vi "Periodic Tasks.vi"(8 "error in":errorcluster) -> ()   [LabVIEW 2020]
doc: "This VI runs in parallel to other tasks. It can contain as many user-defined periodic loops as you need. These can carry out PID or other sorts of timed response."
uses:
  <vilib>/Rock Robotics/WPI/Joystick/XBox Buttons Indexer.ctl
  <vilib>/Rock Robotics/WPI/ThirdParty/JAS_Junk/TrajLib/SlewRateLimiter_New.vi
  <vilib>/Rock Robotics/WPI/ThirdParty/JAS_Junk/TrajLib/SlewRateLimiter_Reset.vi
  <vilib>/Rock Robotics/WPI/ThirdParty/JAS_Junk/TrajLib/SlewRateLimiter_Calculate.vi
  <vilib>/Rock Robotics/WPI/ThirdParty/JAS_Junk/TrajLib/SlewRateLimiter_SetRate.vi
  <vilib>/Rock Robotics/WPI/Utilities/WPI_GetSetVariantRefNum.vi
  Robot Global Data.vi
  <vilib>/Rock Robotics/Network Tables/NT Write Number.vi
  <vilib>/Rock Robotics/WPI/ThirdParty/JAS_Junk/TrajLib/Trajectory_Library.lvlib
panel:
  out "limit 5":bool
  out "limit 4":bool
  out "limit 3":bool
  out "limit 2":bool
  out "limit 1":bool
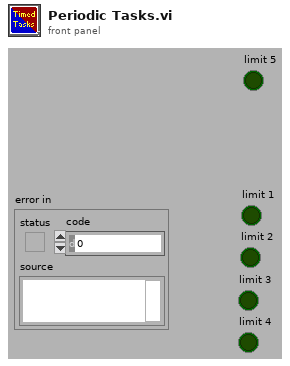
[diagram p1: front panel]
types:
  T1 = typedef "WPI_MotorControlDeviceRef.ctl" = cluster{"DeviceStatus":errorcluster, "Type":T2, "PWM":cluster{"PWM Channel":T3, "DeadBand":T4}, "CAN":cluster{"Device Number":u8, "SetOutput VI Ref":variant, "GetOutput VI Ref":variant, "Enable VI Ref":variant, "Disable VI Ref":variant, "Data":variant}, "Invert":bool, "DIO PWM":cluster{"PWM \"Enable\" Channel":T3, "DIOChannel":T5, "PWM Rate":dbl}}
  T2 = typedef "WPI_MotorControlType.ctl" = enum16{"PWM", "CAN", "DIO PWM"}
  T3 = typedef "FPGA_DIOPWMChannel.ctl" = enum8{"PWM 0", "PWM 1", "PWM 2", "PWM 3", "PWM 4", "PWM 5", "PWM 6", "PWM 7", "PWM 8", "PWM 9", "PWM MXP 0", "PWM MXP 1", "PWM MXP 2", "PWM MXP 3", "PWM MXP 4", "PWM MXP 5", "PWM MXP 6", "PWM MXP 7", "PWM MXP 8", "PWM MXP 9", "Invalid"}
  T4 = typedef "WPI_PWMDeadband.ctl" = cluster{"Name":string, "maxPositivePwm":i32, "minPositivePwm":i32, "centerPwm":i32, "maxNegativePwm":i32, "minNegativePwm":i32, "angularRange":u16}
  T5 = typedef "FPGA_DIOChannel.ctl" = enum8{"DIO 0", "DIO 1", "DIO 2", "DIO 3", "DIO 4", "DIO 5", "DIO 6", "DIO 7", "DIO 8", "DIO 9", "DIO MXP 0", "DIO MXP 1", "DIO MXP 2", "DIO MXP 3", "DIO MXP 4", "DIO MXP 5", "DIO MXP 6", "DIO MXP 7", "DIO MXP 8", "DIO MXP 9", "DIO MXP 10", "DIO MXP 11", "DIO MXP 12", "DIO MXP 13", "DIO MXP 14", "DIO MXP 15", "SPI Port CS1", "SPI Port CS2", "SPI Port CS3", "SPI Port MISO", "SPI Port MOSI", "Invalid"}
  T6 = typedef "WPI_SwitchDevRef.ctl" = cluster{"DevStatus":errorcluster, "DIO Channel":T5, "CntIndex":T7, "Normally Closed":bool}
  T7 = typedef "FPGA_CounterCtrSystemIndex.ctl" = enum8{"Ctr 0", "Ctr 1", "Ctr 2", "Ctr 3", "Ctr 4", "Ctr 5", "Ctr 6", "Ctr 7", "Invalid"}
  T8 = typedef "WPI_GyroDevRef.ctl" = cluster{"DevStatus":errorcluster, "Analog Channel":T9, "Gain (VoltsPerDegree/Second)":dbl, "Gyro Type":enum16{"Analog", "XRS450"}, "Handle":i32, "SPI Bus":T10, "Device Found":bool, "Sample Rate":dbl, "Calibrate On Open":bool, "Offset":dbl}
  T9 = typedef "FPGA_AIChannel.ctl" = enum8{"AI 0", "AI 1", "AI 2", "AI 3", "AI MXP 0", "AI MXP 1", "AI MXP 2", "AI MXP 3", "Invalid"}
  T10 = typedef "spi_bus.ctl" = enum16{"SPI On-Board, CS0", "SPI On-Board, CS1", "SPI On-Board, CS2", "SPI On-Board, CS3", "SPI MXP", "Invalid"}
  T11 = typedef "XBox Buttons Indexer.ctl" = enum16{"A", "B", "X", "Y", "Left Bumper", "Right Bumper", "Back", "Start", "Left Joystick", "Right Joystick"}
  T12 = typedef "Trajectory_Library.lvlib/SWERVE_DRIVE_MODULE_STATE.ctl" = cluster{"Speed":dbl, "Angle":T13}
  T13 = typedef "Trajectory_Library.lvlib/ROTATION2D.ctl" = cluster{"VALUE":dbl, "COS":dbl, "SIN":dbl}
  T14 = typedef "WPI_JoystickDevRef.ctl" = cluster{"Device":T15}
  T15 = typedef "WPI_JoystickDeviceEnum.ctl" = enum16{"USB 0", "USB 1", "USB 2", "USB 3", "USB 4", "USB 5"}
  T16 = typedef "Trajectory_Library.lvlib/SWERVE_DRIVE_MODULE_POSITION.ctl" = cluster{"Distance":dbl, "Angle":T13, "P":bool}
  T17 = typedef "WPI_DriverStationRobotMode2.ctl" = enum16{"Autonomous Disabled", "Autonomous Enabled", "Teleop Disabled", "Teleop Enabled", "Disconnected", "Finish", "Test Disabled", "Test Enabled", "Emergency Stopped"}
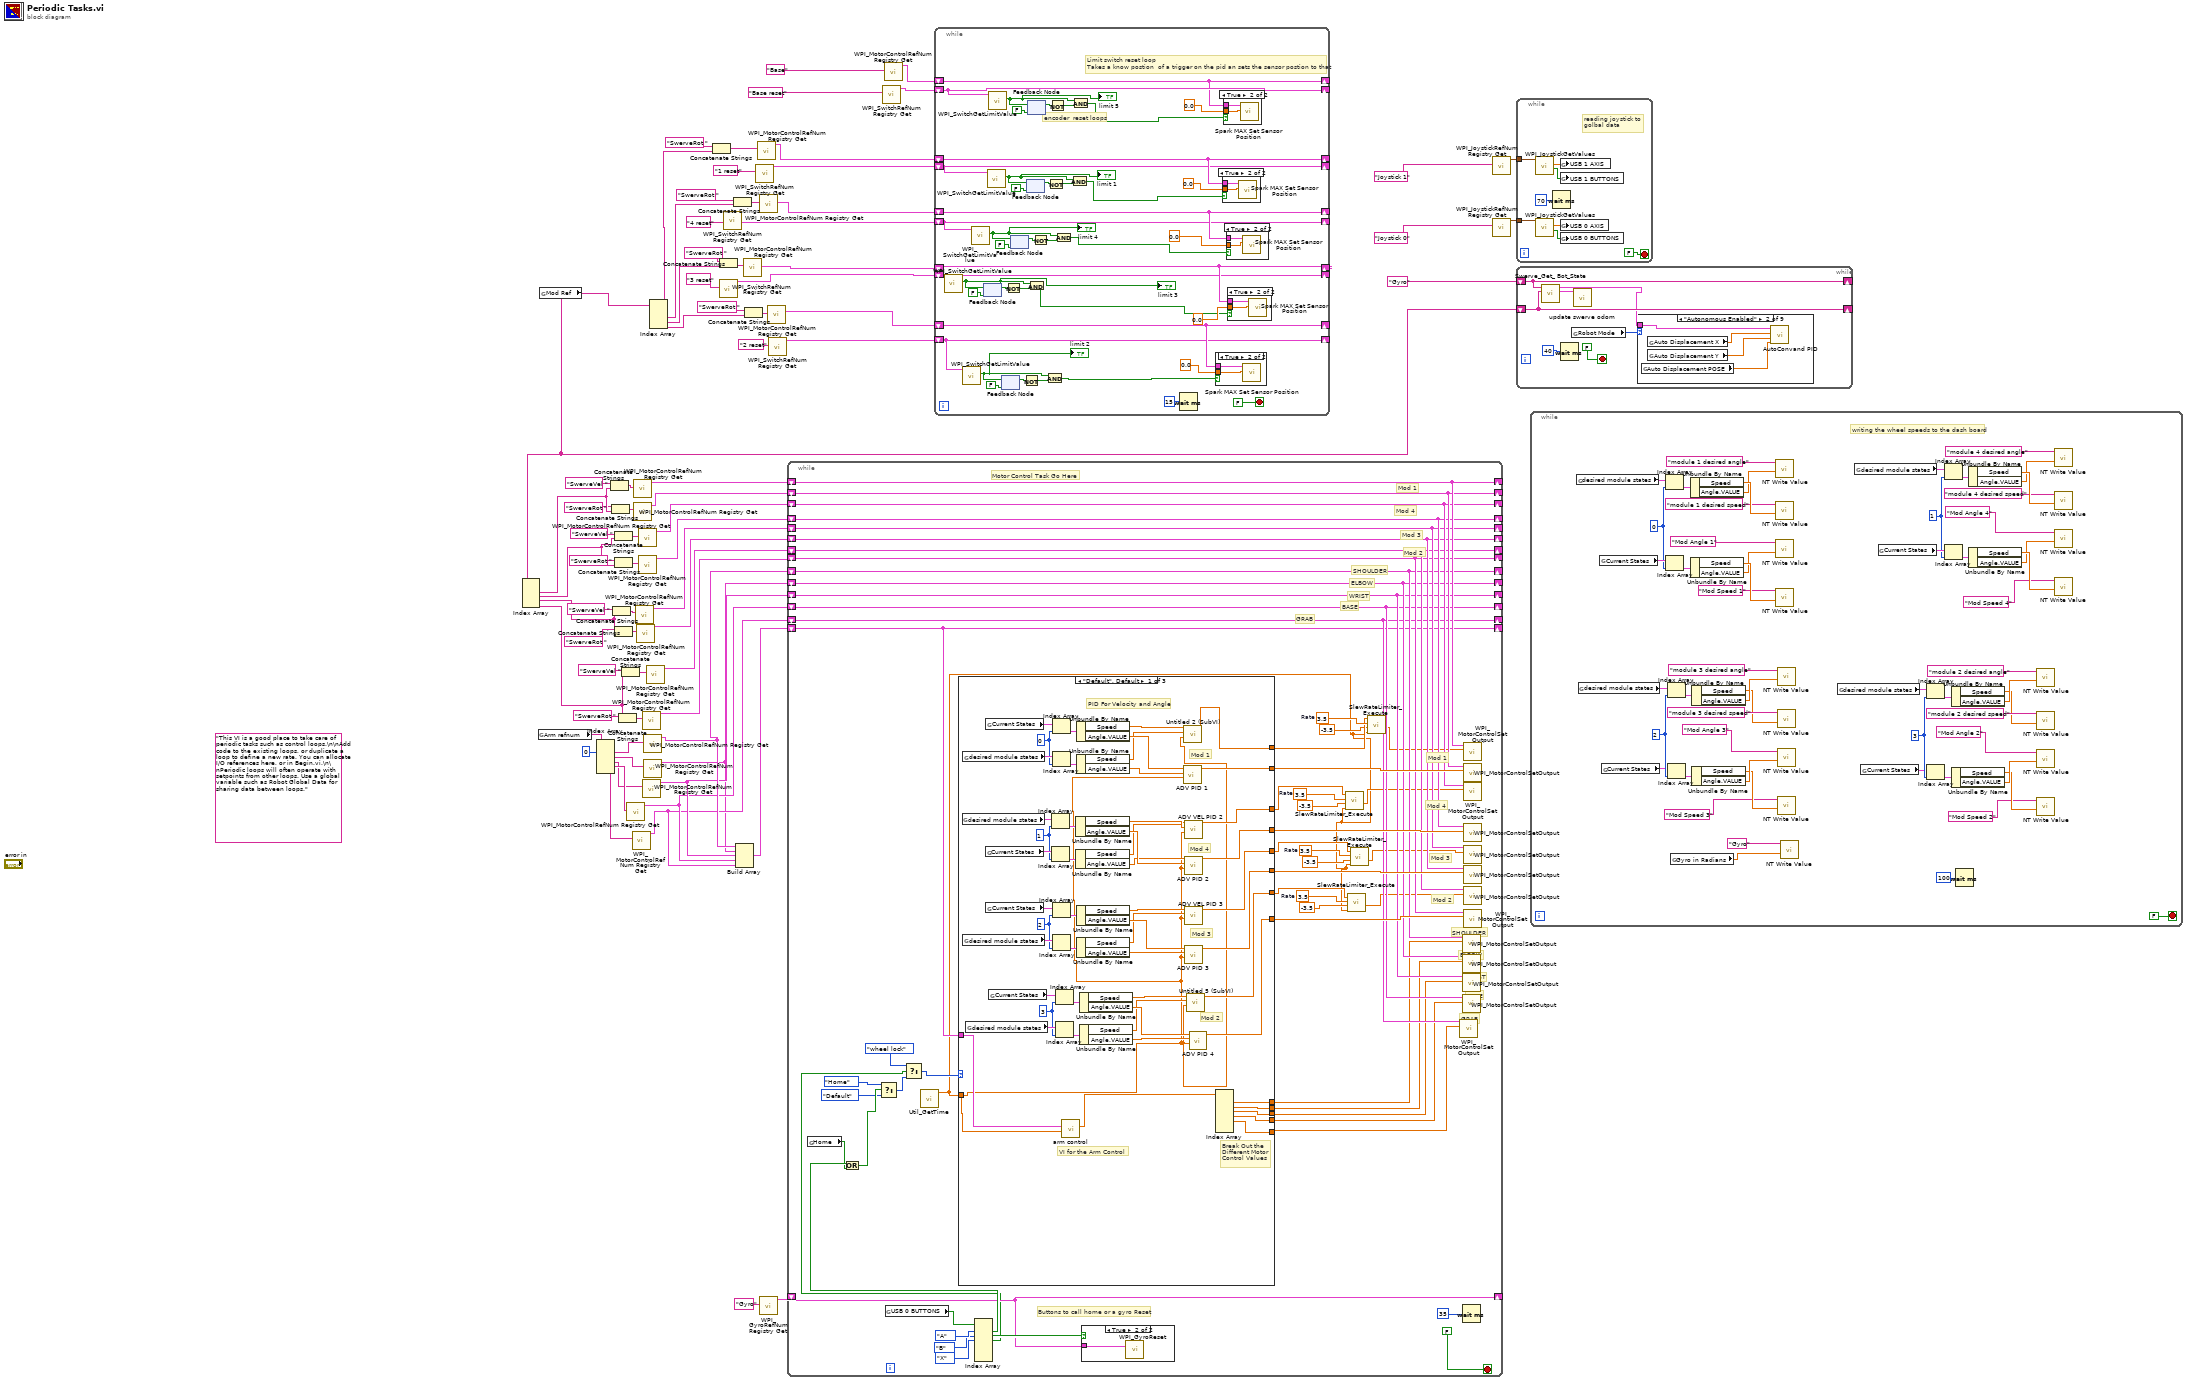
[diagram p0: block diagram]
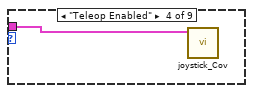
[diagram p4: hidden frame]
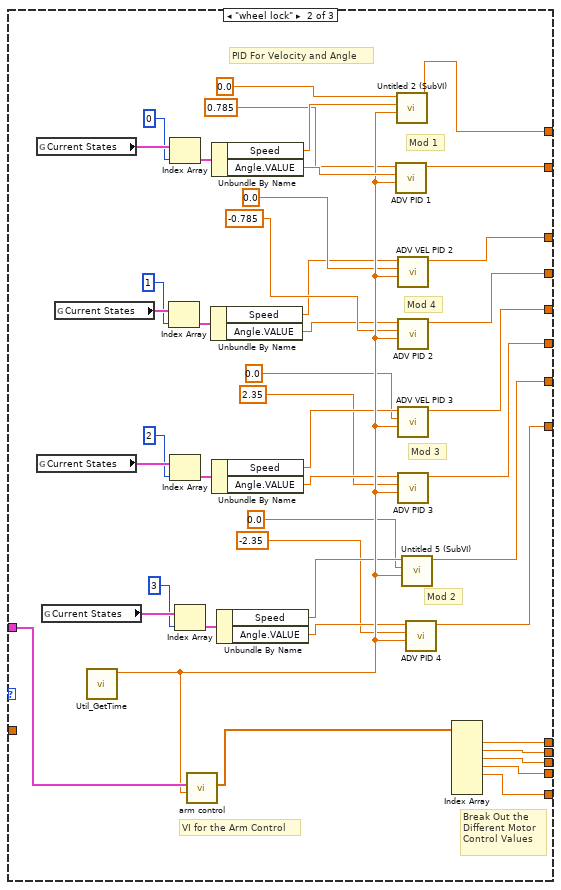
[diagram p10: hidden frame]
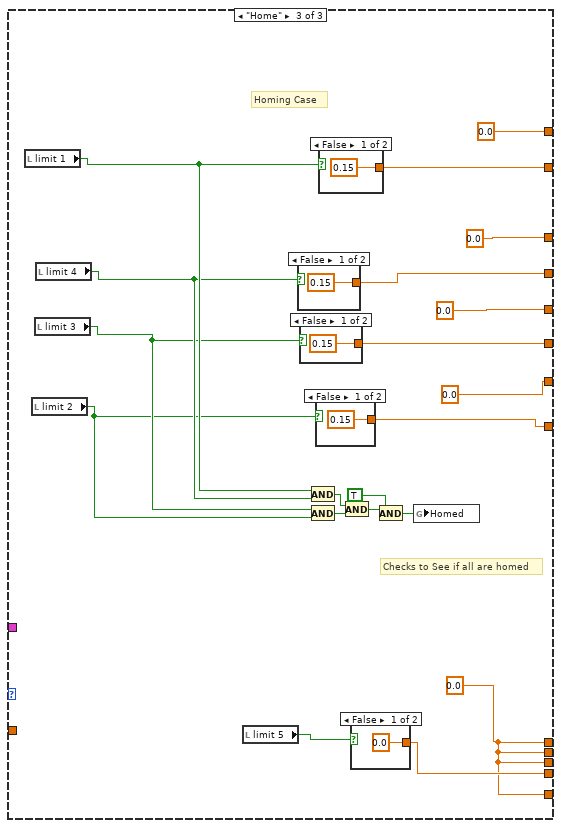
[diagram p11: hidden frame]
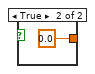
[diagram p12: hidden frame]
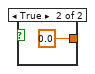
[diagram p13: hidden frame]
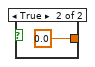
[diagram p14: hidden frame]
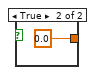
[diagram p15: hidden frame]
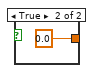
[diagram p16: hidden frame]
diagram:
  (unwired) "This VI is a good place to take care of periodic tasks such as control loops.\n\nAdd code to the existing loops, or duplicate a loop to define a new rate. You can allocate I/O references here, or in Begin.vi.\n\nPeriodic loops will often operate with setpoints from other loops. Use a global variable such as Robot Global Data for sharing data between loops."
  n1 = global read "Robot Global Data.vi" "Arm refnum"() -> (w7:string[])
  n2 = global read "Robot Global Data.vi" "Mod Ref"() -> (w22:string[])
  n3 = Index Array(array=w22) -> (element #1=w35:string, element #2=w40:string, element #3=w49:string, element #4=w50:string)  [unwired: 4 in]
  n4 = Index Array(array=w7, index #1=0 ("index")) -> (element #1=w9:string, element #2=w10:string, element #3=w11:string, element #4=w12:string, element #5=w13:string)  [unwired: 4 in]
  n5 = Concatenate Strings("SwerveVel " ("refnum name"), w35) -> (w32:string)
  n6 = Concatenate Strings("SwerveRot " ("refnum name"), w35) -> (w31:string)
  n7 = Concatenate Strings("SwerveVel " ("refnum name"), w49) -> (w42:string)
  n8 = Concatenate Strings("SwerveVel " ("refnum name"), w40) -> (w38:string)
  n9 = Concatenate Strings("SwerveRot " ("refnum name"), w40) -> (w39:string)
  n10 = Concatenate Strings("SwerveRot " ("refnum name"), w49) -> (w41:string)
  n11 = Concatenate Strings("SwerveRot " ("refnum name"), w50) -> (w48:string)
  n12 = Concatenate Strings("SwerveVel " ("refnum name"), w50) -> (w47:string)
  n13 = call <vilib>:"WPI_MotorControlRefNum Registry Get.vi"("refnum name"=w12) -> ("MotorControlDevRef"=w4:T1)  [unwired: 9 in, 1 out]
  n14 = call <vilib>:"WPI_MotorControlRefNum Registry Get.vi"("refnum name"=w13) -> ("MotorControlDevRef"=w3:T1)  [unwired: 9 in, 1 out]
  n15 = call <vilib>:"WPI_MotorControlRefNum Registry Get.vi"("refnum name"=w32) -> ("MotorControlDevRef"=w30:T1)  [unwired: 9 in, 1 out]
  n16 = call <vilib>:"WPI_MotorControlRefNum Registry Get.vi"("refnum name"=w31) -> ("MotorControlDevRef"=w29:T1)  [unwired: 9 in, 1 out]
  n17 = call <vilib>:"WPI_MotorControlRefNum Registry Get.vi"("refnum name"=w42) -> ("MotorControlDevRef"=w26:T1)  [unwired: 9 in, 1 out]
  n18 = call <vilib>:"WPI_MotorControlRefNum Registry Get.vi"("refnum name"=w41) -> ("MotorControlDevRef"=w25:T1)  [unwired: 9 in, 1 out]
  n19 = call <vilib>:"WPI_MotorControlRefNum Registry Get.vi"("refnum name"=w38) -> ("MotorControlDevRef"=w28:T1)  [unwired: 9 in, 1 out]
  n20 = call <vilib>:"WPI_MotorControlRefNum Registry Get.vi"("refnum name"=w39) -> ("MotorControlDevRef"=w27:T1)  [unwired: 9 in, 1 out]
  n21 = call <vilib>:"WPI_MotorControlRefNum Registry Get.vi"("refnum name"=w48) -> ("MotorControlDevRef"=w23:T1)  [unwired: 9 in, 1 out]
  n22 = call <vilib>:"WPI_MotorControlRefNum Registry Get.vi"("refnum name"=w11) -> ("MotorControlDevRef"=w5:T1)  [unwired: 9 in, 1 out]
  n23 = call <vilib>:"WPI_MotorControlRefNum Registry Get.vi"("refnum name"=w9) -> ("MotorControlDevRef"=w6:T1)  [unwired: 9 in, 1 out]
  n24 = call <vilib>:"WPI_MotorControlRefNum Registry Get.vi"("refnum name"=w10) -> ("MotorControlDevRef"=w2:T1)  [unwired: 9 in, 1 out]
  n25 = call <vilib>:"WPI_MotorControlRefNum Registry Get.vi"("refnum name"=w47) -> ("MotorControlDevRef"=w24:T1)  [unwired: 9 in, 1 out]
  n26 = Index Array(array=w22) -> (element #1=w65:string, element #2=w61:string, element #3=w58:string, element #4=w55:string)  [unwired: 4 in]
  n27 = Concatenate Strings("SwerveRot " ("refnum name"), w65) -> (w64:string)
  n28 = call <vilib>:"WPI_SwitchRefNum Registry Get.vi"("refnum name"="3 reset") -> ("SwitchDevRef"=w72:T6)  [unwired: 9 in, 1 out]
  n29 = Concatenate Strings("SwerveRot " ("refnum name"), w58) -> (w57:string)
  n30 = call <vilib>:"WPI_SwitchRefNum Registry Get.vi"("refnum name"="4 reset") -> ("SwitchDevRef"=w71:T6)  [unwired: 9 in, 1 out]
  n31 = Concatenate Strings("SwerveRot " ("refnum name"), w61) -> (w60:string)
  n32 = Build Array(w6, w2, w5, w4, w3) -> (w1:T1[])
  n33 = call <vilib>:"WPI_MotorControlRefNum Registry Get.vi"("refnum name"=w57) -> ("MotorControlDevRef"=w73:T1)  [unwired: 9 in, 1 out]
  n34 = Concatenate Strings("SwerveRot " ("refnum name"), w55) -> (w54:string)
  n35 = call <vilib>:"WPI_SwitchRefNum Registry Get.vi"("refnum name"="1 reset") -> ("SwitchDevRef"=w66:T6)  [unwired: 9 in, 1 out]
  n36 = call <vilib>:"WPI_MotorControlRefNum Registry Get.vi"("refnum name"=w64) -> ("MotorControlDevRef"=w67:T1)  [unwired: 9 in, 1 out]
  n37 = call <vilib>:"WPI_MotorControlRefNum Registry Get.vi"("refnum name"=w60) -> ("MotorControlDevRef"=w70:T1)  [unwired: 9 in, 1 out]
  n38 = call <vilib>:"WPI_GyroRefNum Registry Get.vi"("refnum name"="Gyro") -> ("GyroDevRef"=w52:T8)  [unwired: 9 in, 1 out]
  n39 = call <vilib>:"WPI_MotorControlRefNum Registry Get.vi"("refnum name"=w54) -> ("MotorControlDevRef"=w76:T1)  [unwired: 9 in, 1 out]
  n40 = call <vilib>:"WPI_SwitchRefNum Registry Get.vi"("refnum name"="2 reset") -> ("SwitchDevRef"=w77:T6)  [unwired: 9 in, 1 out]
  n41 = while {
    shift-right: [w124] -> _
    shift-left: w30 -> [w124]
    shift-right: [w123] -> _
    shift-left: w29 -> [w123]
    shift-right: [w122] -> _
    shift-left: w28 -> [w122]
    shift-right: [w121] -> _
    shift-left: w27 -> [w121]
    shift-right: [w120] -> _
    shift-left: w26 -> [w120]
    shift-right: [w119] -> _
    shift-left: w25 -> [w119]
    shift-right: [w118] -> _
    shift-left: w24 -> [w118]
    shift-right: [w117] -> _
    shift-left: w23 -> [w117]
    shift-right: [w116] -> _
    shift-left: w52 -> [w116]
    shift-right: [w113] -> _
    shift-left: w6 -> [w113]
    shift-right: [w112] -> _
    shift-left: w2 -> [w112]
    shift-right: [w111] -> _
    shift-left: w5 -> [w111]
    shift-right: [w110] -> _
    shift-left: w4 -> [w110]
    shift-right: [w109] -> _
    shift-left: w3 -> [w109]
    shift-right: [w108] -> _
    shift-left: w1 -> [w108]
    stop <- FALSE stop-if-true
    w82 = 3.5  # Rate
    w86 = 3.5  # Rate
    w89 = 3.5  # Rate
    w94 = 3.5  # Rate
    # "Buttons to call home or a gyro Reset"
    # "Mod 4"
    # "Mod 4"
    # "Mod 3"
    # "Mod 3"
    # "Mod 2"
    # "Mod 2"
    # "Mod 1"
    # "Mod 1"
    # "GRAB"
    # "BASE"
    # "WRIST"
    # "ELBOW"
    # "SHOULDER"
    # "BASE"
    # "GRAB"
    # "WRIST"
    # "ELBOW"
    # "SHOULDER"
    # "Motor Control Task Go Here"
    n42 = global read "Robot Global Data.vi" "Home"() -> (w115:bool)
    n43 = global read "Robot Global Data.vi" "USB 0 BUTTONS"() -> (w114:bool[])
    n44 = call <vilib>:"Util_GetTime.vi"() -> ("FPGA_Time_Seconds"=w78:dbl)  [unwired: 9 in, 2 out]
    n45 = Index Array(array=w114, index #1=XBox_Buttons_Indexer."A" ("XBox Buttons"), index #2=XBox_Buttons_Indexer."B" ("XBox Buttons"), index #3=XBox_Buttons_Indexer."X" ("XBox Buttons")) -> (element #1=w125:bool, element #2=w126:bool, element #3=w95:bool)  [unwired: 4 in, 4 out]
    n46 = Or(x=w125, y=w115) -> (x .or. y?=w100:bool)
    n47 = Select(t=enum16{"Default", "Home", "wheel lock"}."Home", s=w100, f=enum16{"Default", "Home", "wheel lock"}."Default") -> (s? t:f=w102:enum16{"Default", "Home", "wheel lock"})
    n48 = Select(t=enum16{"Default", "Home", "wheel lock"}."wheel lock", s=w95, f=w102) -> (s? t:f=w101:enum16{"Default", "Home", "wheel lock"})
    n49 = case shown="\"Default\", Default" w101 {
      tunnel: [w154 w213 0.0] -> w93
      tunnel: [w151 w211 0.0] -> w88
      tunnel: [w145 w209 0.0] -> w83
      tunnel: [w148 w210 0.0] -> w80
      tunnel: [w186 w230 w249] -> w132
      tunnel: [w185 w229 w243] -> w131
      tunnel: [w184 w228 w245] -> w130
      tunnel: [w183 w227 w247] -> w129
      tunnel: w108 -> [w144 w208 _]
      tunnel: [w142 w206 w235] -> w107
      tunnel: [w141 w205 w235] -> w104
      tunnel: [w140 w204 w235] -> w106
      tunnel: [w139 w203 w236] -> w103
      tunnel: [w138 w202 w235] -> w105
      tunnel: w78 -> [w135 _ _]
      frame "Default", Default {
        w165 = 0 ("index")
        w164 = 1 ("index")
        w163 = 2 ("index")
        w172 = 3 ("index")
        # "Mod 2"
        # "Mod 3"
        # "Mod 4"
        # "Mod 1"
        # "Break Out the\nDifferent Motor\nControl Values"
        # "VI for the Arm Control"
        # "PID For Velocity and Angle"
        n50 = global read "Robot Global Data.vi" "desired module states"() -> (w169:T12[])
        n51 = global read "Robot Global Data.vi" "desired module states"() -> (w167:T12[])
        n52 = global read "Robot Global Data.vi" "desired module states"() -> (w171:T12[])
        n53 = global read "Robot Global Data.vi" "desired module states"() -> (w174:T12[])
        n54 = global read "Robot Global Data.vi" "Current States"() -> (w177:T12[])
        n55 = global read "Robot Global Data.vi" "Current States"() -> (w176:T12[])
        n56 = global read "Robot Global Data.vi" "Current States"() -> (w180:T12[])
        n57 = global read "Robot Global Data.vi" "Current States"() -> (w181:T12[])
        n58 = Index Array(array=w169, index=w164) -> (element=w168:T12)
        n59 = Index Array(array=w177, index=w164) -> (element=w178:T12)
        n60 = Index Array(array=w176, index=w165) -> (element=w175:T12)
        n61 = Index Array(array=w167, index=w165) -> (element=w166:T12)
        n62 = Index Array(array=w180, index=w163) -> (element=w179:T12)
        n63 = Index Array(array=w171, index=w163) -> (element=w170:T12)
        n64 = Index Array(array=w181, index=w172) -> (element=w182:T12)
        n65 = Index Array(array=w174, index=w172) -> (element=w173:T12)
        n66 = call "arm control.vi"("FPGA_Time_Seconds"=w135, "appended array"=w144) -> ("appended array 2"=w143:dbl[])  [unwired: 9 in]
        n67 = Unbundle By Name(w168) -> ("Speed"=w137:dbl, "Angle.VALUE"=w160:dbl)
        n68 = Unbundle By Name(w178) -> ("Speed"=w136:dbl, "Angle.VALUE"=w159:dbl)
        n69 = Unbundle By Name(w175) -> ("Speed"=w153:dbl, "Angle.VALUE"=w161:dbl)
        n70 = Unbundle By Name(w166) -> ("Speed"=w152:dbl, "Angle.VALUE"=w162:dbl)
        n71 = Unbundle By Name(w179) -> ("Speed"=w150:dbl, "Angle.VALUE"=w157:dbl)
        n72 = Unbundle By Name(w170) -> ("Speed"=w149:dbl, "Angle.VALUE"=w158:dbl)
        n73 = Unbundle By Name(w182) -> ("Speed"=w147:dbl, "Angle.VALUE"=w155:dbl)
        n74 = Unbundle By Name(w173) -> ("Speed"=w146:dbl, "Angle.VALUE"=w156:dbl)
        n75 = call "ADV PID 1.vi"("Time"=w135, "SP-SetPoint"=w162, "PV-Measurement"=w161) -> ("CO-ControlOutput"=w186:dbl)  [unwired: 8 in]
        n76 = call "Untitled 2 (SubVI).vi"("Time"=w135, "SP-SetPoint"=w152, "PV-Measurement"=w153) -> ("CO-ControlOutput"=w154:dbl)  [unwired: 8 in]
        n77 = call "ADV VEL PID 2.vi"("Time"=w135, "SP-SetPoint"=w137, "PV-Measurement"=w136) -> ("CO-ControlOutput"=w151:dbl)  [unwired: 8 in]
        n78 = call "ADV PID 2.vi"("Time"=w135, "SP-SetPoint in"=w160, "PV-Measurement in"=w159) -> ("CO-ControlOutput"=w183:dbl)  [unwired: 8 in]
        n79 = call "ADV VEL PID 3.vi"("Time"=w135, "SP-SetPoint"=w149, "PV-Measurement"=w150) -> ("CO-ControlOutput"=w145:dbl)  [unwired: 8 in]
        n80 = call "ADV PID 3.vi"("Time in"=w135, "SP-SetPoint 3"=w158, "PV-Measurement 3"=w157) -> ("CO-ControlOutput"=w184:dbl)  [unwired: 8 in]
        n81 = call "Untitled 5 (SubVI).vi"("Time"=w135, "SP-SetPoint"=w146, "PV-Measurement"=w147) -> ("CO-ControlOutput"=w148:dbl)  [unwired: 8 in]
        n82 = call "ADV PID 4.vi"("Time in"=w135, "SP-SetPoint 4"=w156, "PV-Measurement 4"=w155) -> ("CO-ControlOutput"=w185:dbl)  [unwired: 8 in]
        n83 = Index Array(array=w143) -> (element #1=w142:dbl, element #2=w141:dbl, element #3=w140:dbl, element #4=w139:dbl, element #5=w138:dbl)  [unwired: 7 in, 2 out]
      }
      frame "wheel lock" {
        # "Mod 2"
        # "Mod 3"
        # "Mod 4"
        # "Mod 1"
        # "Break Out the\nDifferent Motor\nControl Values"
        # "VI for the Arm Control"
        # "PID For Velocity and Angle"
        n84 = global read "Robot Global Data.vi" "Current States"() -> (w219:T12[])
        n85 = global read "Robot Global Data.vi" "Current States"() -> (w221:T12[])
        n86 = global read "Robot Global Data.vi" "Current States"() -> (w224:T12[])
        n87 = global read "Robot Global Data.vi" "Current States"() -> (w225:T12[])
        n88 = call <vilib>:"Util_GetTime.vi"() -> ("FPGA_Time_Seconds"=w201:dbl)  [unwired: 9 in, 2 out]
        n89 = Index Array(array=w225, index=1) -> (element=w226:T12)
        n90 = Index Array(array=w219, index=0) -> (element=w218:T12)
        n91 = Index Array(array=w221, index=2) -> (element=w220:T12)
        n92 = Index Array(array=w224, index=3) -> (element=w223:T12)
        n93 = call "arm control.vi"("FPGA_Time_Seconds"=w201, "appended array"=w208) -> ("appended array 2"=w207:dbl[])  [unwired: 9 in]
        n94 = Unbundle By Name(w226) -> ("Speed"=w195:dbl, "Angle.VALUE"=w196:dbl)
        n95 = Unbundle By Name(w218) -> ("Speed"=w212:dbl, "Angle.VALUE"=w214:dbl)
        n96 = Unbundle By Name(w220) -> ("Speed"=w194:dbl, "Angle.VALUE"=w193:dbl)
        n97 = Unbundle By Name(w223) -> ("Speed"=w190:dbl, "Angle.VALUE"=w189:dbl)
        n98 = call "ADV PID 1.vi"("Time"=w201, "SP-SetPoint"=w214, "PV-Measurement"=0.785) -> ("CO-ControlOutput"=w230:dbl)  [unwired: 8 in]
        n99 = call "Untitled 2 (SubVI).vi"("Time"=w201, "SP-SetPoint"=w212, "PV-Measurement"=0.0) -> ("CO-ControlOutput"=w213:dbl)  [unwired: 8 in]
        n100 = call "ADV VEL PID 2.vi"("Time"=w201, "SP-SetPoint"=0.0 ("PV-Measurement"), "PV-Measurement"=w195) -> ("CO-ControlOutput"=w211:dbl)  [unwired: 8 in]
        n101 = call "ADV PID 2.vi"("Time"=w201, "SP-SetPoint in"=-0.785 ("PV-Measurement"), "PV-Measurement in"=w196) -> ("CO-ControlOutput"=w227:dbl)  [unwired: 8 in]
        n102 = call "ADV VEL PID 3.vi"("Time"=w201, "SP-SetPoint"=0.0 ("PV-Measurement"), "PV-Measurement"=w194) -> ("CO-ControlOutput"=w209:dbl)  [unwired: 8 in]
        n103 = call "ADV PID 3.vi"("Time in"=w201, "SP-SetPoint 3"=2.35 ("PV-Measurement"), "PV-Measurement 3"=w193) -> ("CO-ControlOutput"=w228:dbl)  [unwired: 8 in]
        n104 = call "Untitled 5 (SubVI).vi"("Time"=w201, "SP-SetPoint"=0.0 ("PV-Measurement"), "PV-Measurement"=w190) -> ("CO-ControlOutput"=w210:dbl)  [unwired: 8 in]
        n105 = call "ADV PID 4.vi"("Time in"=w201, "SP-SetPoint 4"=-2.35 ("PV-Measurement"), "PV-Measurement 4"=w189) -> ("CO-ControlOutput"=w229:dbl)  [unwired: 8 in]
        n106 = Index Array(array=w207) -> (element #1=w206:dbl, element #2=w205:dbl, element #3=w204:dbl, element #4=w203:dbl, element #5=w202:dbl)  [unwired: 7 in, 2 out]
      }
      frame "Home" {
        w235 = 0.0
        # "Checks to See if all are homed"
        # "Homing Case"
        n107 = local read "limit 1"() -> (w240:bool)
        n108 = local read "limit 2"() -> (w237:bool)
        n109 = local read "limit 3"() -> (w238:bool)
        n110 = local read "limit 4"() -> (w239:bool)
        n111 = local read "limit 5"() -> (w233:bool)
        n112 = case shown="False" w239 {
          tunnel: [0.15 ("CO-ControlOutput") 0.0 ("CO-ControlOutput")] -> w247
          frame False {
          }
          frame True {
          }
        }
        n113 = case shown="False" w238 {
          tunnel: [0.15 ("CO-ControlOutput") 0.0 ("CO-ControlOutput")] -> w245
          frame False {
          }
          frame True {
          }
        }
        n114 = And(x=w240, y=w239) -> (x .and. y?=w242:bool)
        n115 = And(x=w238, y=w237) -> (x .and. y?=w241:bool)
        n116 = case shown="False" w237 {
          tunnel: [0.15 ("CO-ControlOutput") 0.0 ("CO-ControlOutput")] -> w243
          frame False {
          }
          frame True {
          }
        }
        n117 = case shown="False" w240 {
          tunnel: [0.15 ("CO-ControlOutput") 0.0 ("CO-ControlOutput")] -> w249
          frame False {
          }
          frame True {
          }
        }
        n118 = And(x=w242, y=w241) -> (x .and. y?=w234:bool)
        n119 = case shown="False" w233 {
          tunnel: [0.0 ("CO-ControlOutput") 0.0 ("CO-ControlOutput")] -> w236
          frame False {
          }
          frame True {
          }
        }
        n120 = And(x=w234, y=TRUE) -> (x .and. y?=w232:bool)
        n121 = global write "Robot Global Data.vi" "Homed"(w232) -> ()
      }
    }
    n122 = case shown="True" w126 {
      tunnel: w116 -> [_ w261]
      frame False {
      }
      frame True {
        n123 = call <vilib>:"WPI_GyroReset.vi"("GyroDevRef"=w261) -> ()  [unwired: 9 in, 2 out]
      }
    }
    n124 = call <vilib>:"SlewRateLimiter_Execute.vi"("Time"=w78, "NegativeRate"=-3.5, "PositiveRate"=w89, "Input"=w88) -> ("Output"=w87:dbl)  [unwired: 6 in, 1 out]
    n125 = call <vilib>:"SlewRateLimiter_Execute.vi"("Time"=w78, "NegativeRate"=-3.5, "PositiveRate"=w82, "Input"=w80) -> ("Output"=w81:dbl)  [unwired: 6 in, 1 out]
    n126 = call <vilib>:"SlewRateLimiter_Execute.vi"("Time"=w78, "NegativeRate"=-3.5, "PositiveRate"=w86, "Input"=w83) -> ("Output"=w84:dbl)  [unwired: 6 in, 1 out]
    n127 = call <vilib>:"SlewRateLimiter_Execute.vi"("Time"=w78, "NegativeRate"=-3.5, "PositiveRate"=w94, "Input"=w93) -> ("Output"=w91:dbl)  [unwired: 6 in, 1 out]
    n128 = call <vilib>:"WPI_MotorControlSetOutput.vi"("Output"=w105, "MotorControlDevRef"=w109) -> ()  [unwired: 7 in, 3 out]
    n129 = call <vilib>:"WPI_MotorControlSetOutput.vi"("Output"=w107, "MotorControlDevRef"=w113) -> ()  [unwired: 7 in, 3 out]
    n130 = call <vilib>:"WPI_MotorControlSetOutput.vi"("Output"=w104, "MotorControlDevRef"=w112) -> ()  [unwired: 7 in, 3 out]
    n131 = call <vilib>:"WPI_MotorControlSetOutput.vi"("Output"=w103, "MotorControlDevRef"=w110) -> ()  [unwired: 7 in, 3 out]
    n132 = Wait (ms)(milliseconds to wait=u32 35) -> ()  [unwired: 1 out]
    n133 = call <vilib>:"WPI_MotorControlSetOutput.vi"("Output"=w106, "MotorControlDevRef"=w111) -> ()  [unwired: 7 in, 3 out]
    n134 = call <vilib>:"WPI_MotorControlSetOutput.vi"("Output"=w91, "MotorControlDevRef"=w124) -> ()  [unwired: 7 in, 3 out]
    n135 = call <vilib>:"WPI_MotorControlSetOutput.vi"("Output"=w132, "MotorControlDevRef"=w123) -> ()  [unwired: 7 in, 3 out]
    n136 = call <vilib>:"WPI_MotorControlSetOutput.vi"("Output"=w87, "MotorControlDevRef"=w122) -> ()  [unwired: 7 in, 3 out]
    n137 = call <vilib>:"WPI_MotorControlSetOutput.vi"("Output"=w129, "MotorControlDevRef"=w121) -> ()  [unwired: 7 in, 3 out]
    n138 = call <vilib>:"WPI_MotorControlSetOutput.vi"("Output"=w84, "MotorControlDevRef"=w120) -> ()  [unwired: 7 in, 3 out]
    n139 = call <vilib>:"WPI_MotorControlSetOutput.vi"("Output"=w130, "MotorControlDevRef"=w119) -> ()  [unwired: 7 in, 3 out]
    n140 = call <vilib>:"WPI_MotorControlSetOutput.vi"("Output"=w81, "MotorControlDevRef"=w118) -> ()  [unwired: 7 in, 3 out]
    n141 = call <vilib>:"WPI_MotorControlSetOutput.vi"("Output"=w131, "MotorControlDevRef"=w117) -> ()  [unwired: 7 in, 3 out]
  }
  n142 = call <vilib>:"WPI_SwitchRefNum Registry Get.vi"("refnum name"="Base reset") -> ("SwitchDevRef"=w15:T6)  [unwired: 9 in, 1 out]
  n143 = call <vilib>:"WPI_MotorControlRefNum Registry Get.vi"("refnum name"="Base") -> ("MotorControlDevRef"=w17:T1)  [unwired: 9 in, 1 out]
  n144 = while {
    shift-right: [w301] -> _
    shift-left: w67 -> [w301]
    shift-right: [w300] -> _
    shift-left: w66 -> [w300]
    shift-right: [w299] -> _
    shift-left: w70 -> [w299]
    shift-right: [w298] -> _
    shift-left: w71 -> [w298]
    shift-right: [w297] -> _
    shift-left: w73 -> [w297]
    shift-right: [w296] -> _
    shift-left: w72 -> [w296]
    shift-right: [w295] -> _
    shift-left: w76 -> [w295]
    shift-right: [w294] -> _
    shift-left: w77 -> [w294]
    shift-right: [w262] -> _
    shift-left: w17 -> [w262]
    shift-right: [w263] -> _
    shift-left: w15 -> [w263]
    stop <- FALSE stop-if-true
    # "Limit switch reset loop\nTakes a know postion  of a trigger on the pid an sets the sensor postion to that"
    # "encoder  reset loops"
    n145 = call <vilib>:"WPI_SwitchGetLimitValue.vi"("SwitchDevRef"=w296) -> ("Switch Pressed"=w271:bool)  [unwired: 8 in, 2 out]
    "limit 3" <- w271
    n146 = call <vilib>:"WPI_SwitchGetLimitValue.vi"("SwitchDevRef"=w294) -> ("Switch Pressed"=w270:bool)  [unwired: 8 in, 2 out]
    "limit 2" <- w270
    n147 = call <vilib>:"WPI_SwitchGetLimitValue.vi"("SwitchDevRef"=w298) -> ("Switch Pressed"=w273:bool)  [unwired: 8 in, 2 out]
    "limit 4" <- w273
    n148 = feedback #1(FALSE ("Switch Pressed")) -> (w286:bool)
    n149 = feedback-in #1(w271) -> ()
    n150 = call <vilib>:"WPI_SwitchGetLimitValue.vi"("SwitchDevRef"=w300) -> ("Switch Pressed"=w274:bool)  [unwired: 8 in, 2 out]
    "limit 1" <- w274
    n151 = call <vilib>:"WPI_SwitchGetLimitValue.vi"("SwitchDevRef"=w263) -> ("Switch Pressed"=w269:bool)  [unwired: 8 in, 2 out]
    "limit 5" <- w269
    n152 = feedback #2(FALSE ("Switch Pressed")) -> (w283:bool)
    n153 = feedback-in #2(w270) -> ()
    n154 = Not(x=w286) -> (.not. x?=w285:bool)
    n155 = feedback #3(FALSE ("Switch Pressed")) -> (w289:bool)
    n156 = feedback-in #3(w273) -> ()
    n157 = Not(x=w283) -> (.not. x?=w284:bool)
    n158 = feedback-in #4(w274) -> ()
    n159 = feedback #4(FALSE ("Switch Pressed")) -> (w292:bool)
    n160 = feedback #5(FALSE ("Switch Pressed")) -> (w265:bool)
    n161 = feedback-in #5(w269) -> ()
    n162 = And(x=w271, y=w285) -> (x .and. y?=w272:bool)
    n163 = Not(x=w289) -> (.not. x?=w290:bool)
    n164 = And(x=w270, y=w284) -> (x .and. y?=w275:bool)
    n165 = Not(x=w292) -> (.not. x?=w291:bool)
    n166 = Not(x=w265) -> (.not. x?=w266:bool)
    n167 = And(x=w273, y=w290) -> (x .and. y?=w276:bool)
    n168 = And(x=w274, y=w291) -> (x .and. y?=w277:bool)
    n169 = And(x=w269, y=w266) -> (x .and. y?=w268:bool)
    n170 = Wait (ms)(milliseconds to wait=u32 15) -> ()  [unwired: 1 out]
    n171 = case shown="True" w275 {
      tunnel: w295 -> [_ w313]
      tunnel: 0.0 ("2") -> [_ w312]
      frame False {
      }
      frame True {
        n172 = call <vilib>:"Spark MAX Set Sensor Position.vi"("Position"=w312, "MotorControlDeviceRef"=w313) -> ()  [unwired: 8 in, 2 out]
      }
    }
    n173 = case shown="True" w277 {
      tunnel: w301 -> [_ w307]
      tunnel: 0.0 ("1") -> [_ w306]
      frame False {
      }
      frame True {
        n174 = call <vilib>:"Spark MAX Set Sensor Position.vi"("Position"=w306, "MotorControlDeviceRef"=w307) -> ()  [unwired: 8 in, 2 out]
      }
    }
    n175 = case shown="True" w268 {
      tunnel: w262 -> [_ w305]
      tunnel: 0.0 ("1") -> [_ w304]
      frame False {
      }
      frame True {
        n176 = call <vilib>:"Spark MAX Set Sensor Position.vi"("Position"=w304, "MotorControlDeviceRef"=w305) -> ()  [unwired: 8 in, 2 out]
      }
    }
    n177 = case shown="True" w276 {
      tunnel: w299 -> [_ w309]
      tunnel: 0.0 ("4") -> [_ w308]
      frame False {
      }
      frame True {
        n178 = call <vilib>:"Spark MAX Set Sensor Position.vi"("Position"=w308, "MotorControlDeviceRef"=w309) -> ()  [unwired: 8 in, 2 out]
      }
    }
    n179 = case shown="True" w272 {
      tunnel: w297 -> [_ w311]
      tunnel: 0.0 ("3") -> [_ w310]
      frame False {
      }
      frame True {
        n180 = call <vilib>:"Spark MAX Set Sensor Position.vi"("Position"=w310, "MotorControlDeviceRef"=w311) -> ()  [unwired: 8 in, 2 out]
      }
    }
  }
  n181 = call <vilib>:"WPI_JoystickRefNum Registry Get.vi"("refnum name"="Joystick 1") -> ("JoystickDevRef"=w19:T14)  [unwired: 1 in, 9 out]
  n182 = call <vilib>:"WPI_JoystickRefNum Registry Get.vi"("refnum name"="Joystick 0") -> ("JoystickDevRef"=w18:T14)  [unwired: 1 in, 9 out]
  n183 = while {
    tunnel: w19 -> [w315]
    tunnel: w18 -> [w314]
    stop <- FALSE stop-if-true
    # "reading joystick to \ngolbal data"
    n184 = call <vilib>:"WPI_JoystickGetValues.vi"("JoystickDevRef"=w315) -> ("Buttons"=w318:bool[], "Axes"=w319:dbl[])  [unwired: 6 in, 3 out]
    n185 = call <vilib>:"WPI_JoystickGetValues.vi"("JoystickDevRef"=w314) -> ("Buttons"=w317:bool[], "Axes"=w316:dbl[])  [unwired: 6 in, 3 out]
    n186 = Wait (ms)(milliseconds to wait=u32 70) -> ()  [unwired: 1 out]
    n187 = global write "Robot Global Data.vi" "USB 1 AXIS"(w319) -> ()
    n188 = global write "Robot Global Data.vi" "USB 1 BUTTONS"(w318) -> ()
    n189 = global write "Robot Global Data.vi" "USB 0 AXIS"(w316) -> ()
    n190 = global write "Robot Global Data.vi" "USB 0 BUTTONS"(w317) -> ()
  }
  n191 = while {
    shift-right: [w326] -> _
    shift-left: "Gyro" ("refnum name") -> [w326]
    shift-right: [w324] -> _
    shift-left: w22 -> [w324]
    stop <- FALSE stop-if-true
    n192 = call "Swerve_Get_ Bot_State.vi"("Mod Ref"=w324, "refnum name"=w326) -> ("Mod Pos"=w328:T16[], "Mod State"=w323:T12[])  [unwired: 8 in]
    n193 = Wait (ms)(milliseconds to wait=u32 40) -> ()  [unwired: 1 out]
    n194 = global read "Robot Global Data.vi" "Robot Mode"() -> (w322:T17)
    n195 = call "update swerve odom.vi"("Module Pos"=w328) -> ()  [unwired: 11 in]
    n196 = case shown="\"Autonomous Enabled\"" w322 {
      tunnel: w323 -> [_ w332 _ w333 _ _ _ _ _]
      frame "Autonomous Disabled", Default {
      }
      frame "Autonomous Enabled" {
        n197 = global read "Robot Global Data.vi" "Auto Displacement POSE"() -> (w329:dbl)
        n198 = global read "Robot Global Data.vi" "Auto Displacement X"() -> (w331:dbl)
        n199 = global read "Robot Global Data.vi" "Auto Displacement Y"() -> (w330:dbl)
        n200 = call "AutoConvand PID.vi"("Rot SetPoint"=w329, "Y SetPiont"=w330, "X SetPoint"=w331, "Mod State"=w332) -> ()  [unwired: 8 in]
      }
      frame "Teleop Disabled" {
      }
      frame "Teleop Enabled" {
        n201 = call "joystick_Cov.vi"("Mod State"=w333) -> ()  [unwired: 11 in]
      }
      frame "Disconnected" {
      }
      frame "Finish" {
      }
      frame "Test Disabled" {
      }
      frame "Test Enabled" {
      }
      frame "Emergency Stopped" {
      }
    }
  }
  n202 = while {
    stop <- FALSE stop-if-true
    w349 = 3 ("index")
    w362 = 1 ("index")
    w371 = 2 ("index")
    w385 = 0 ("index")
    # "writing the wheel speeds to the dash board"
    n203 = global read "Robot Global Data.vi" "desired module states"() -> (w387:T12[])
    n204 = global read "Robot Global Data.vi" "desired module states"() -> (w369:T12[])
    n205 = global read "Robot Global Data.vi" "Current States"() -> (w389:T12[])
    n206 = global read "Robot Global Data.vi" "Current States"() -> (w367:T12[])
    n207 = Index Array(array=w387, index=w385) -> (element=w386:T12)
    n208 = Index Array(array=w389, index=w385) -> (element=w388:T12)
    n209 = Index Array(array=w369, index=w371) -> (element=w370:T12)
    n210 = Index Array(array=w367, index=w371) -> (element=w368:T12)
    n211 = global read "Robot Global Data.vi" "Gyro in Radians"() -> (w341:dbl)
    n212 = Unbundle By Name(w386) -> ("Speed"=w382:dbl, "Angle.VALUE"=w381:dbl)
    n213 = Unbundle By Name(w388) -> ("Speed"=w384:dbl, "Angle.VALUE"=w383:dbl)
    n214 = Unbundle By Name(w370) -> ("Speed"=w374:dbl, "Angle.VALUE"=w375:dbl)
    n215 = Unbundle By Name(w368) -> ("Speed"=w372:dbl, "Angle.VALUE"=w373:dbl)
    n216 = call-poly <vilib>:"NT Write Value.vi"("value"=w381, "name"="module 1 desired angle") -> ()  [unwired: 9 in, 1 out]
    n217 = call-poly <vilib>:"NT Write Value.vi"("value"=w382, "name"="module 1 desired speed") -> ()  [unwired: 9 in, 1 out]
    n218 = call-poly <vilib>:"NT Write Value.vi"("value"=w383, "name"="Mod Angle 1") -> ()  [unwired: 9 in, 1 out]
    n219 = call-poly <vilib>:"NT Write Value.vi"("value"=w384, "name"="Mod Speed 1") -> ()  [unwired: 9 in, 1 out]
    n220 = call-poly <vilib>:"NT Write Value.vi"("value"=w375, "name"="module 3 desired angle") -> ()  [unwired: 9 in, 1 out]
    n221 = call-poly <vilib>:"NT Write Value.vi"("value"=w374, "name"="module 3 desired speed") -> ()  [unwired: 9 in, 1 out]
    n222 = call-poly <vilib>:"NT Write Value.vi"("value"=w373, "name"="Mod Angle 3") -> ()  [unwired: 9 in, 1 out]
    n223 = call-poly <vilib>:"NT Write Value.vi"("value"=w372, "name"="Mod Speed 3") -> ()  [unwired: 9 in, 1 out]
    n224 = call-poly <vilib>:"NT Write Value.vi"("value"=w341, "name"="Gyro") -> ()  [unwired: 9 in, 1 out]
    n225 = global read "Robot Global Data.vi" "desired module states"() -> (w347:T12[])
    n226 = global read "Robot Global Data.vi" "desired module states"() -> (w364:T12[])
    n227 = global read "Robot Global Data.vi" "Current States"() -> (w345:T12[])
    n228 = global read "Robot Global Data.vi" "Current States"() -> (w366:T12[])
    n229 = Index Array(array=w347, index=w349) -> (element=w348:T12)
    n230 = Index Array(array=w345, index=w349) -> (element=w346:T12)
    n231 = Index Array(array=w364, index=w362) -> (element=w363:T12)
    n232 = Index Array(array=w366, index=w362) -> (element=w365:T12)
    n233 = Unbundle By Name(w348) -> ("Speed"=w352:dbl, "Angle.VALUE"=w353:dbl)
    n234 = Unbundle By Name(w346) -> ("Speed"=w350:dbl, "Angle.VALUE"=w351:dbl)
    n235 = Wait (ms)(milliseconds to wait=u32 100) -> ()  [unwired: 1 out]
    n236 = Unbundle By Name(w363) -> ("Speed"=w359:dbl, "Angle.VALUE"=w358:dbl)
    n237 = Unbundle By Name(w365) -> ("Speed"=w361:dbl, "Angle.VALUE"=w360:dbl)
    n238 = call-poly <vilib>:"NT Write Value.vi"("value"=w353, "name"="module 2 desired angle") -> ()  [unwired: 9 in, 1 out]
    n239 = call-poly <vilib>:"NT Write Value.vi"("value"=w352, "name"="module 2 desired speed") -> ()  [unwired: 9 in, 1 out]
    n240 = call-poly <vilib>:"NT Write Value.vi"("value"=w351, "name"="Mod Angle 2") -> ()  [unwired: 9 in, 1 out]
    n241 = call-poly <vilib>:"NT Write Value.vi"("value"=w350, "name"="Mod Speed 2") -> ()  [unwired: 9 in, 1 out]
    n242 = call-poly <vilib>:"NT Write Value.vi"("value"=w358, "name"="module 4 desired angle") -> ()  [unwired: 9 in, 1 out]
    n243 = call-poly <vilib>:"NT Write Value.vi"("value"=w359, "name"="module 4 desired speed") -> ()  [unwired: 9 in, 1 out]
    n244 = call-poly <vilib>:"NT Write Value.vi"("value"=w360, "name"="Mod Angle 4") -> ()  [unwired: 9 in, 1 out]
    n245 = call-poly <vilib>:"NT Write Value.vi"("value"=w361, "name"="Mod Speed 4") -> ()  [unwired: 9 in, 1 out]
  }
